vi "datasetRid.get.vi"(8 "error in (no error)":errorcluster, 11 "Stream in":refnum<class "Stream.lvclass">) -> (0 "error out":errorcluster, 2 "Dataset RID":string, 3 "Stream out":refnum<class "Stream.lvclass">)   [LabVIEW 2020, in "Nominal Streaming.lvlib" / "Stream.lvclass"]
uses:
  Stream.lvclass
  Stream.lvclass/Stream.ctl
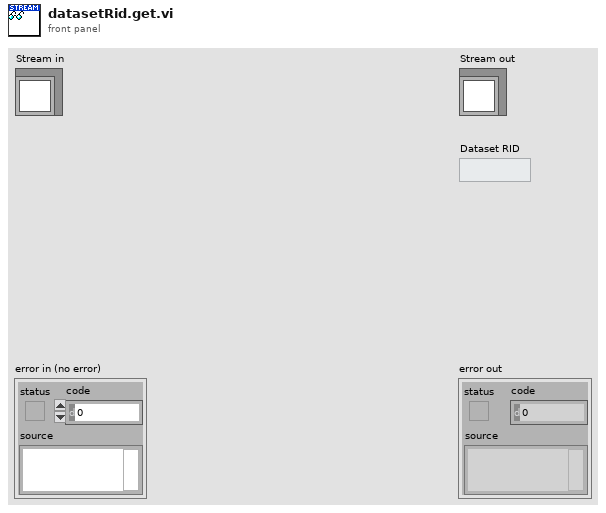
[diagram p1: front panel]
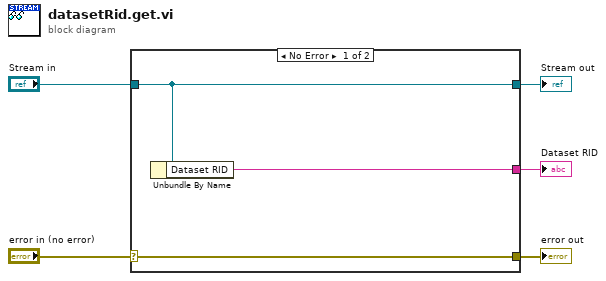
[diagram p0: block diagram]
diagram:
  n1 = case shown="No Error" "error in (no error)" {
    selector: "error in (no error)" -> [w8 w9]
    tunnel: [w8 w9] -> w4
    tunnel: [w7 w10] -> w2
    tunnel: "Stream in" -> [w7 w10]
    tunnel: [w6 _] -> w1
    frame No Error {
      n2 = Unbundle By Name(w7) -> ("Dataset RID"=w6:string)
    }
    frame Error {
    }
  }
  "error out" <- w4
  "Stream out" <- w2
  "Dataset RID" <- w1
